vi "Create Tree Shortcut Menu.vi"(9 "Selection type":T1, 11 "Menu in":refnum<k9>) -> (0 "error out":errorcluster)   [LabVIEW 2019, in "Panther Dashboard.lvlib"]
uses:
  Panther Dashboard.lvlib
  Selection Type--enum.ctl
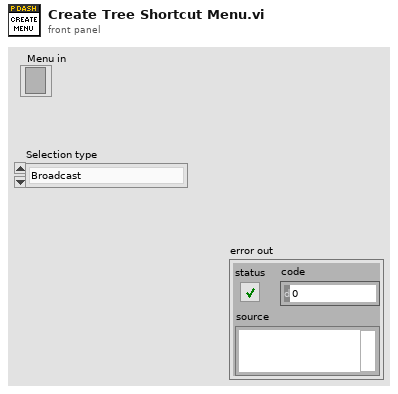
[diagram p1: front panel]
types:
  T1 = typedef "Panther Dashboard.lvlib/Selection Type--enum.ctl" = enum16{"Broadcast", "Request", "Module", "Public API"}
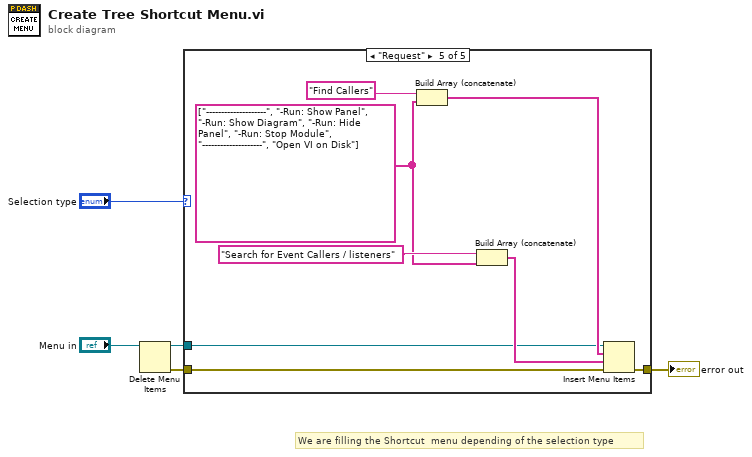
[diagram p0: block diagram]
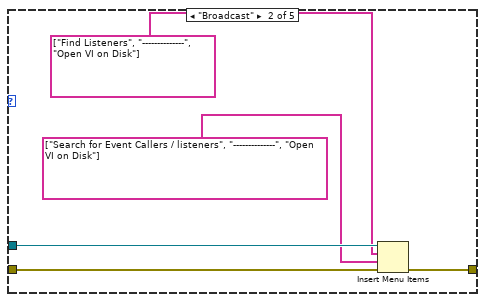
[diagram p3: hidden frame]
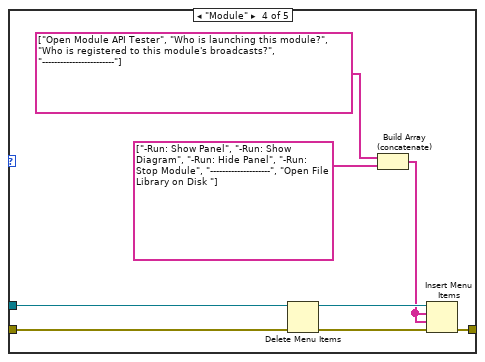
[diagram p5: hidden frame]
diagram:
  # "We are filling the Shortcut  menu depending of the selection type"
  n1 = Delete Menu Items(9:"Menu in") -> (0:w4:errorcluster, 3:w1:refnum<k9>)  [unwired: 3 in]
  n2 = case shown="\"Request\"" "Selection type" {
    tunnel: [w6 w11 w12 w19 w28] -> w5
    tunnel: w4 -> [w6 w10 w12 w18 w27]
    tunnel: w1 -> [_ w9 _ w13 w22]
    frame Default {
    }
    frame "Broadcast" {
      n3 = Insert Menu Items(6:w10, 7:string[] ["Search for Event Callers / listeners", "--------------", "Open VI on Disk"], 8:string[] ["Find Listeners", "--------------", "Open VI on Disk"], 9:w9) -> (0:w11:errorcluster)  [unwired: 2 in, 2 out]
    }
    frame "Public API" {
    }
    frame "Module" {
      n4 = Delete Menu Items(6:w18, 9:w13) -> (0:w20:errorcluster, 3:w17:refnum<k9>)  [unwired: 2 in]
      n5 = Build Array (concatenate)(string[] ["Open Module API Tester", "Who is launching this module?", "Who is registered to this module's broadcasts?", "------------------------"] ("item names"), string[] ["-Run: Show Panel", "-Run: Show Diagram", "-Run: Hide Panel", "-Run: Stop Module", "--------------------", "Open File Library on Disk "] ("item names")) -> (w14:string[])
      n6 = Insert Menu Items(6:w20, 7:w14, 8:w14, 9:w17) -> (0:w19:errorcluster)  [unwired: 2 in, 2 out]
    }
    frame "Request" {
      w21 = string[] ["--------------------", "-Run: Show Panel", "-Run: Show Diagram", "-Run: Hide Panel", "-Run: Stop Module", "--------------------", "Open VI on Disk"] ("item names")
      n7 = Build Array (concatenate)("Find Callers", w21) -> (w24:string[])
      n8 = Build Array (concatenate)("Search for Event Callers / listeners", w21) -> (w25:string[])
      n9 = Insert Menu Items(6:w27, 7:w25, 8:w24, 9:w22) -> (0:w28:errorcluster)  [unwired: 2 in, 2 out]
    }
  }
  "error out" <- w5
